vi "Add Bitfile Dependancy.vi"(8 "error in (no error)":errorcluster, 10 "Path":path, 11 "Item Ref in":T1 format="%.0x") -> (0 "error out":errorcluster, 3 "Item Ref out":T1 format="%.0x")   [LabVIEW 2016, in "FPGA Addon System Explorer.lvlib"]
uses:
  FPGA Addon System Explorer.lvlib
  <vilib>/NI Veristand/Custom Device API/Custom Device Item Ref.ctl
  <vilib>/NI Veristand/Custom Device API/Dependent File Optional Info.ctl
  <vilib>/NI Veristand/Custom Device API/Set Item Property (Dependent File).vi
  Shared/Constants.vi
  <vilib>/NI VeriStand/Custom Device API/Custom Device API.lvlib
  Shared/FPGA Addon Shared.lvlib
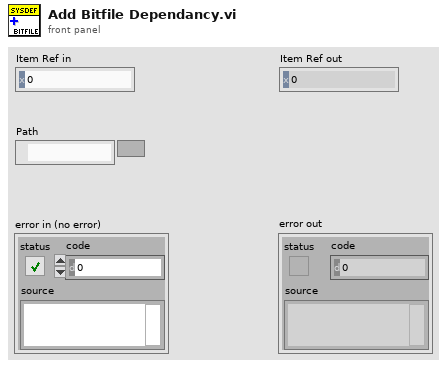
[diagram p1: front panel]
types:
  T1 = typedef "Custom Device API.lvlib/Custom Device Item Ref.ctl" = u64
  T2 = typedef "Custom Device API.lvlib/Dependent File Optional Info.ctl" = cluster{"Version":string, "RTDestination":path, "ForceDownload":bool, "SupportedTarget":string, "MD5":string}
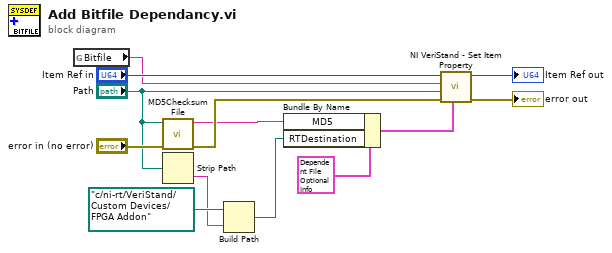
[diagram p0: block diagram]
diagram:
  n1 = global read "Constants.vi" "Bitfile"() -> (w5:string)
  n2 = call <vilib>:"MD5Checksum File.vi"("error in (no error)"="error in (no error)", "Path"="Path") -> ("error out"=w11:errorcluster, "MD5 message-digest"=w10:string)  [unwired: 8 in]
  n3 = Strip Path(path="Path") -> (name=w2:string)  [unwired: 1 out]
  n4 = Build Path(base path=path "c:/ni-rt/VeriStand/Custom Devices/FPGA Addon" ("RTDestination"), name or relative path=w2) -> (appended path=w1:path)
  n5 = Bundle By Name(cluster=T2 {"Version"="1.0", "RTDestination"=path "c:/ni-rt/VeriStand/Custom Devices/FPGA Addon", "ForceDownload"=FALSE, "SupportedTarget"="All", "MD5"=""} ("OptionalInfo"), "MD5"=w10, "RTDestination"=w1) -> (w9:T2)
  n6 = call-poly <vilib>:"NI VeriStand - Set Item Property.vi"("OptionalInfo"=w9, "error in (no error)"=w11, "Path"="Path", "Property Name"=w5, "Item Ref in"="Item Ref in") -> ("error out"=→"error out":errorcluster, "Item Ref out"=→"Item Ref out":T1)  [unwired: 4 in, 1 out]
